vi "Write Dynamic Stop.vi"(8 "error in (no error)":errorcluster, 10 "Dynamic Stop":refnum<user-event>, 11 "Thread in":refnum<class "Thread.lvclass">) -> (0 "error out":errorcluster, 3 "Thread out":refnum<class "Thread.lvclass">)   [LabVIEW 2019, in "Architecture.lvlib" / "Thread.lvclass"]
uses:
  Thread.lvclass
  Thread.lvclass/Thread.ctl
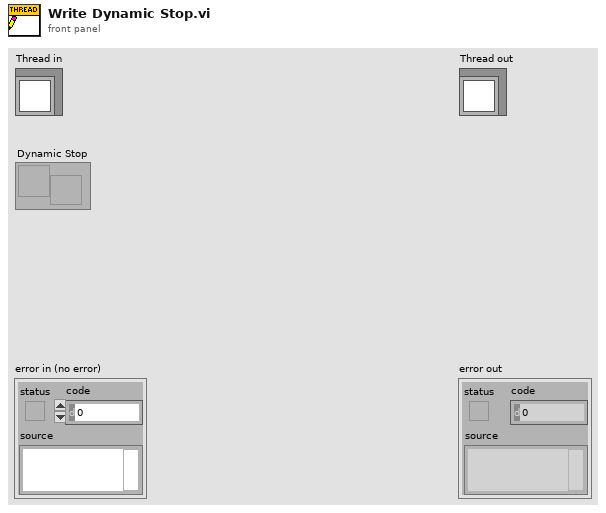
[diagram p1: front panel]
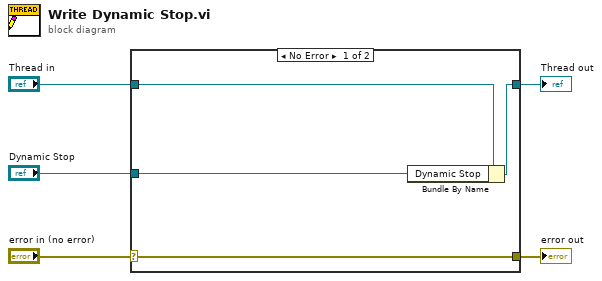
[diagram p0: block diagram]
diagram:
  n1 = case shown="No Error" "error in (no error)" {
    selector: "error in (no error)" -> [w9 w10]
    tunnel: [w9 w10] -> w4
    tunnel: [w7 w11] -> w2
    tunnel: "Thread in" -> [w8 w11]
    tunnel: "Dynamic Stop" -> [w6 _]
    frame No Error {
      n2 = Bundle By Name(cluster=w8, "Dynamic Stop"=w6) -> (w7:refnum<class "Thread.lvclass">)
    }
    frame Error {
    }
  }
  "error out" <- w4
  "Thread out" <- w2
